vi "Load Firmware Data.vi"(8 "Error In":errorcluster, 9 "Firmware Index":i32, 10 "Device Index":i32, 11 "Family Index":i32) -> (0 "Error Out":errorcluster, 1 "Upload Type":string[](array[string]), 2 "Firmware Interface":T1, 3 "Firmware Description":string)   [LabVIEW 2014, in "LMH-LINX.lvlib"]
doc: "Load specified firmware readme."
uses:
  LMH-LINX.lvlib
  Device/Type Defs/Firmware Interface.ctl
  Type Defs/All Firmware Data FGV States.ctl
panel:
  in  "Device Family":u16(ring) items=["National Instruments", "Digilent", "Arduino"]
  in  "Device Type":u16(ring) items=["chipKIT Uno32", "chipKIT uC32", "chipKIT Max32", "chipKIT DP32"]
  in  "Firmware Version":u16(ring) items=["LINX -  Serial / USB", "LINX -  Serial / USB [Debug] "]
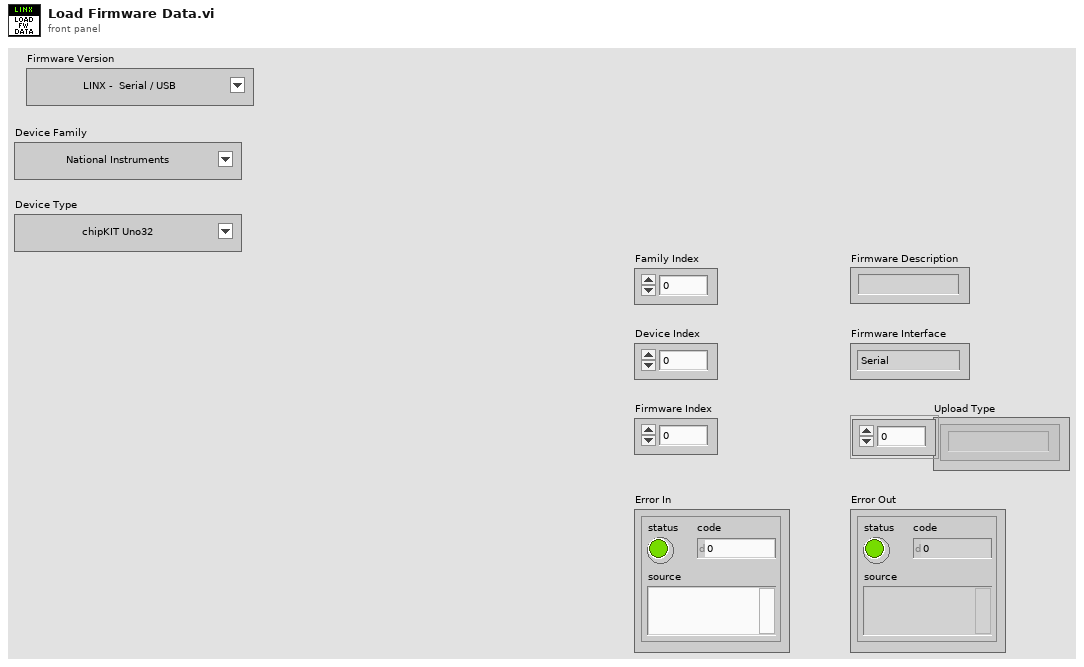
[diagram p1: front panel]
types:
  T1 = typedef "LMH-LINX.lvlib/Firmware Interface.ctl" = enum32{"Serial ", "Ethernet", "WIFI"}
  T2 = typedef "LMH-LINX.lvlib/All Firmware Data FGV States.ctl" = enum16{"Set", "Get"}
  T3 = typedef "LMH-LINX.lvlib/Device Firmware.ctl" = cluster{"Firmware Name":string, "Firmware Path":path, "Description":string, "LINX Interface":string, "Flash Util Working Dir":path, "Flash Util Name":string, "Flash Util Args":string, "Flash Timeout (ms)":i32, "Pre-Built Firmware":string, "Build with Arduino IDE":string}
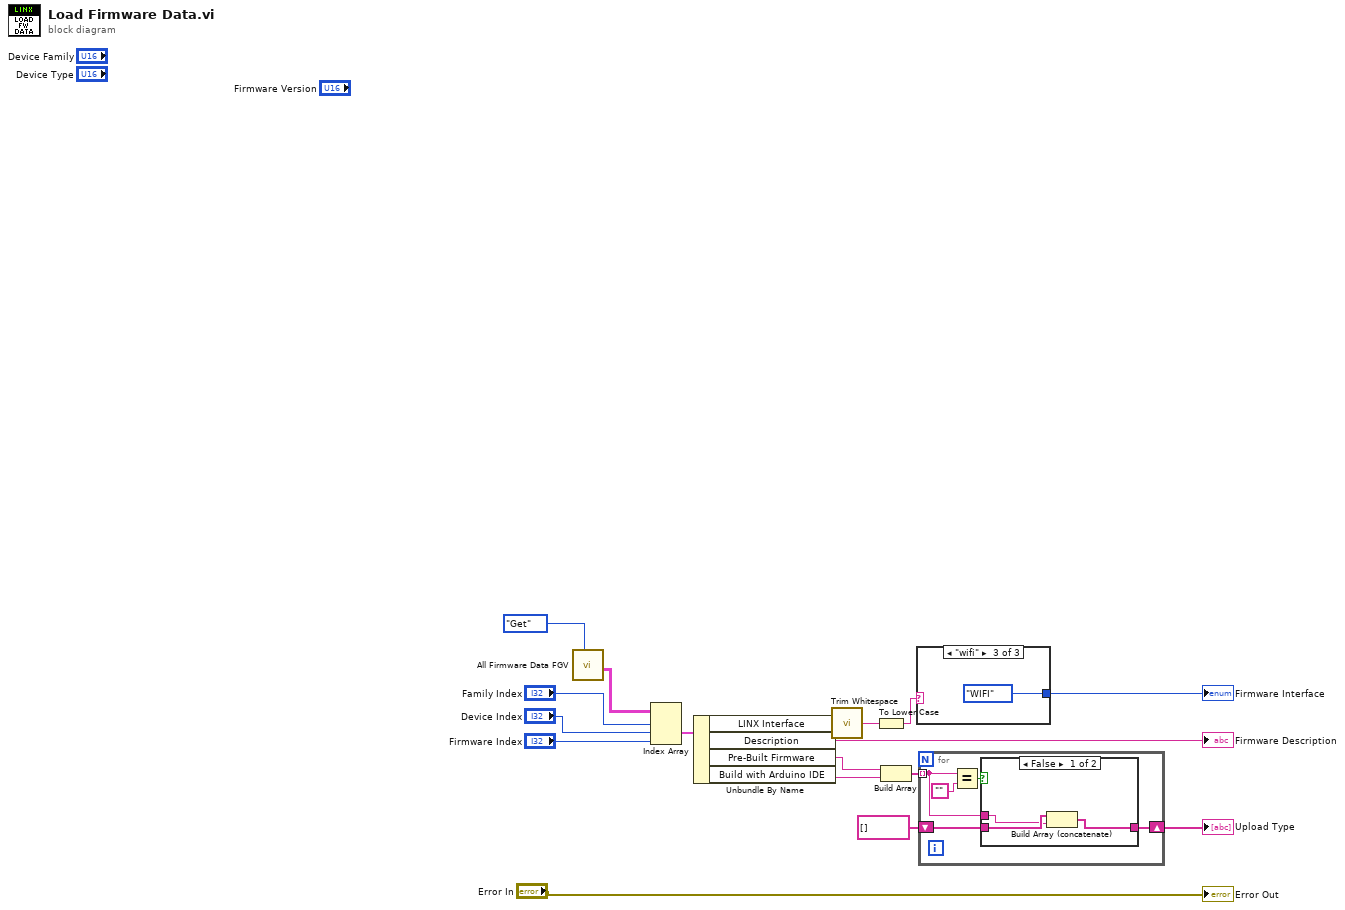
[diagram p0: block diagram]
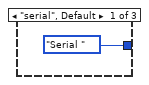
[diagram p3: hidden frame]
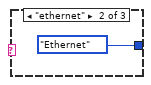
[diagram p4: hidden frame]
diagram:
  n1 = call "All Firmware Data FGV.vi"("All Firmware Data FGV States"=All_Firmware_Data_FGV_States."Get") -> ("Firmwares"=w16:T3[][][])  [unwired: 7 in, 3 out]
  n2 = Index Array(array=w16, index (dim 0)="Family Index", index (dim 1)="Device Index", index (dim 2)="Firmware Index") -> (element=w15:T3)
  n3 = Unbundle By Name(w15) -> ("LINX Interface"=w7:string, "Description"=→"Firmware Description":string, "Pre-Built Firmware"=w5:string, "Build with Arduino IDE"=w4:string)
  n4 = call <vilib>:"Trim Whitespace.vi"("string"=w7) -> ("trimmed string"=w10:string)  [unwired: 1 in]
  n5 = To Lower Case(string=w10) -> (all lower case string=w9:string)
  n6 = Build Array(w5, w4) -> (w3:string[])
  n7 = case shown="\"wifi\"" w9 {
    tunnel: [Firmware_Interface."Serial " ("Firmware Interface") Firmware_Interface."Ethernet" ("Firmware Interface") Firmware_Interface."WIFI" ("Firmware Interface")] -> w8
    frame "serial", Default {
    }
    frame "ethernet" {
    }
    frame "wifi" {
    }
  }
  "Firmware Interface" <- w8
  n8 = for {
    tunnel: w3 -> [w23] mode=indexing
    shift-right: [w22] -> w1
    shift-left: string[] [] -> [w21]
    n9 = Equal?(x=w23, y="") -> (x = y?=w24:bool)
    n10 = case shown="False" w24 {
      tunnel: w23 -> [w26 _]
      tunnel: [w28 w29] -> w22
      tunnel: w21 -> [w27 w29]
      frame False {
        n11 = Build Array (concatenate)(w27, w26) -> (w28:string[])
      }
      frame True {
      }
    }
  }
  "Upload Type" <- w1
  "Error Out" <- "Error In"
